vi "RetrieveValue.vi"(8 "Desired Angle Input":dbl, 9 "Intercept":dbl[](array[numeric]), 10 "Slope":dbl[](array[numeric]), 11 "Angles/Indicies":dbl[](array[numeric])) -> (3 "Value Output":dbl)   [LabVIEW 2012]
doc: "This VI uses the line parameters generated by GenerateLines.vi in order to translate an inputted angle into the value correstponding to that angle. Assuming GenerateLines.vi gives correct output, this function should work for any angle input 0-360 degrees."
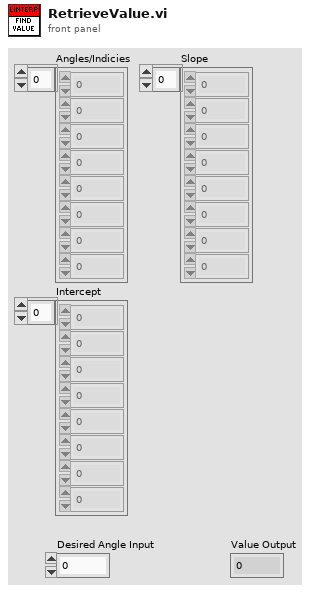
[diagram p1: front panel]
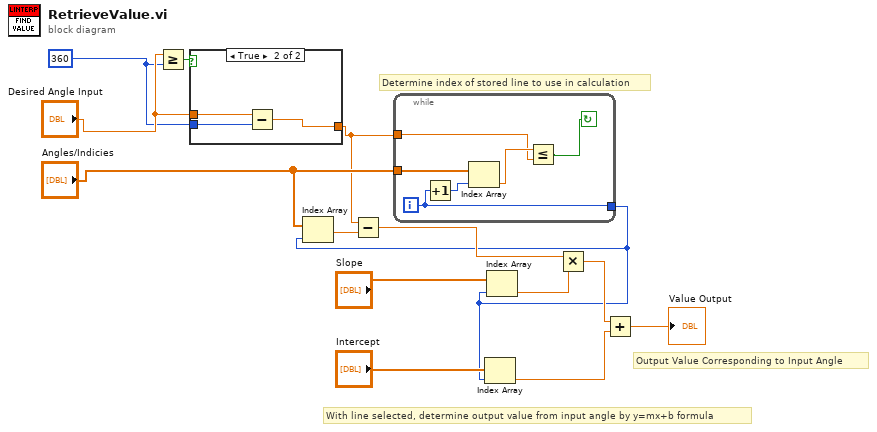
[diagram p0: block diagram]
diagram:
  w2 = 360
  # "Output Value Corresponding to Input Angle"
  # "With line selected, determine output value from input angle by y=mx+b formula"
  # "Determine index of stored line to use in calculation"
  n1 = Greater Or Equal?(x="Desired Angle Input", y=w2) -> (x >= y?=w4:bool)
  n2 = case shown="True" w4 {
    tunnel: "Desired Angle Input" -> [w15 w17]
    tunnel: w2 -> [_ w18]
    tunnel: [w15 w16] -> w1
    frame False {
    }
    frame True {
      n3 = Subtract(x=w17, y=w18) -> (x-y=w16:dbl)
    }
  }
  n4 = while {
    tunnel: "Angles/Indicies" -> [w24]
    tunnel: w1 -> [w21]
    tunnel: [w20] -> w7
    i -> [w20]
    stop <- w23 continue-if-true
    n5 = Increment(x=w20) -> (x+1=w19:i32)
    n6 = Index Array(array=w24, index=w19) -> (element=w22:dbl)
    n7 = Less Or Equal?(x=w22, y=w21) -> (x <= y?=w23:bool)
  }
  n8 = Index Array(array="Angles/Indicies", index=w7) -> (element=w5:dbl)
  n9 = Subtract(x=w1, y=w5) -> (x-y=w9:dbl)
  n10 = Index Array(array="Intercept", index=w7) -> (element=w8:dbl)
  n11 = Index Array(array="Slope", index=w7) -> (element=w12:dbl)
  n12 = Multiply(x=w9, y=w12) -> (x*y=w11:dbl)
  n13 = Add(x=w11, y=w8) -> (x+y=→"Value Output":dbl)
